vi "Exponential_MA.vi"(1 "Input Array":dbl[](array[numeric]), 2 "a":dbl=1.0 min=0.0 max=1.0) -> (0 "Output Array":dbl[](array[numeric]))   [LabVIEW 2023]
uses:
  <vilib>/Analysis/2dsp.llb/1D Convolution (DBL).vi
  <vilib>/Analysis/NI_AALPro.lvlib
panel:
  out "Exponential Window":dbl[](array[numeric])
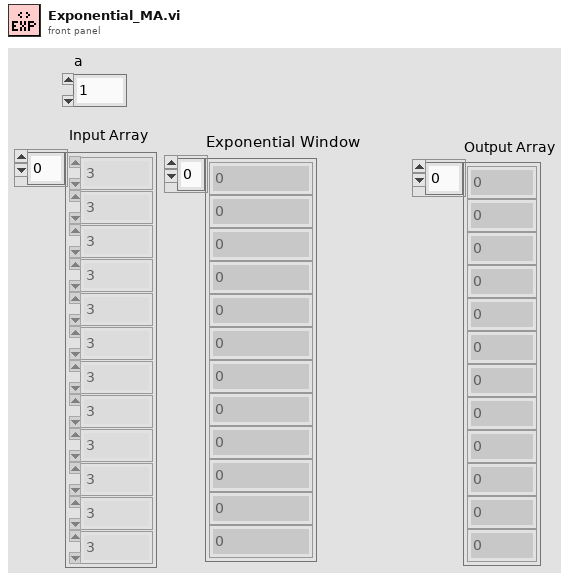
[diagram p1: front panel]
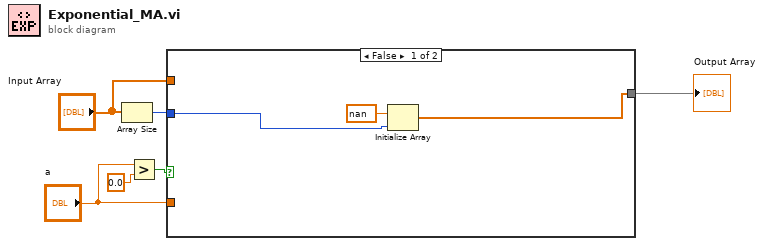
[diagram p0: block diagram]
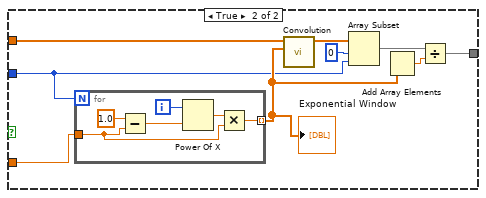
[diagram p2: hidden frame]
diagram:
  n1 = Array Size(array="Input Array") -> (size(s)=w4:i32)
  n2 = Greater?(x="a", y=0.0) -> (0:w3:bool)
  n3 = case shown="False" w3 {
    tunnel: "Input Array" -> [_ w18]
    tunnel: [w7 w13] -> w5
    tunnel: w4 -> [w8 w11]
    tunnel: "a" -> [_ w10]
    frame False {
      n4 = Initialize Array(nan, w8) -> (w7:dbl[])
    }
    frame True {
      n5 = for {
        N: w11 -> [_]
        tunnel: w10 -> [w20]
        tunnel: [w19] -> w12 mode=indexing
        i -> [w22]
        n6 = Subtract(x=1.0, y=w20) -> (x-y=w23:dbl)
        n7 = Power Of X(1:w23, 2:w22) -> (0:w21:dbl)
        n8 = Multiply(x=w21, y=w20) -> (x*y=w19:dbl)
      }
      "Exponential Window" <- w12
      n9 = call-poly <vilib>:"Convolution.vi"("Y"=w12, "X"=w18) -> ("X * Y"=w17:dbl[])  [unwired: 8 in, 1 out]
      n10 = Array Subset(array=w17, index=0, length=w11) -> (w15:dbl[])
      n11 = Add Array Elements(numeric array=w12) -> (sum=w14:dbl)
      n12 = Divide(x=w15, y=w14) -> (x/y=w13:dbl[])
    }
  }
  "Output Array" <- w5
